vi "Constructor.vi"(8 "error in (no error)":errorcluster, 11 "Singleton.lvclass In":refnum<class "Singleton.lvclass">) -> (0 "error out":errorcluster, 3 "SingletonDVR Out":refnum<data-value>)   [LabVIEW 2013, in "Singleton.lvclass"]
uses:
  Singleton.lvclass
  Singleton.lvclass/Singleton.ctl
panel:
  # "SingletonConstructor"
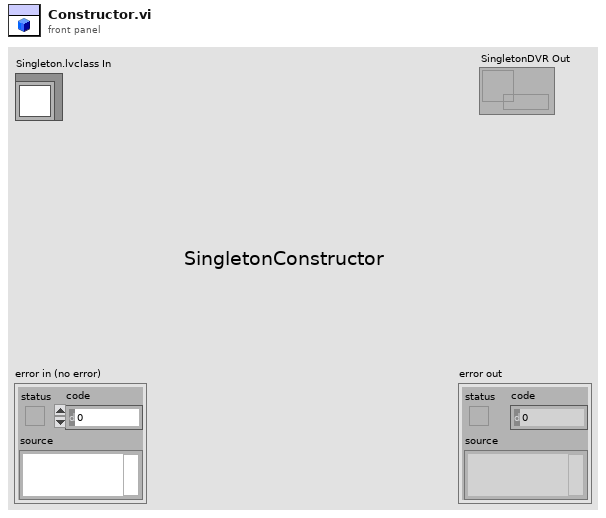
[diagram p1: front panel]
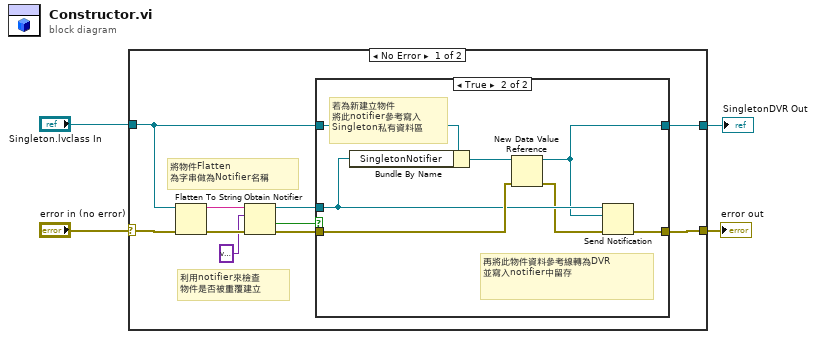
[diagram p0: block diagram]
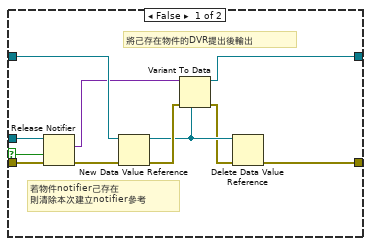
[diagram p2: hidden frame]
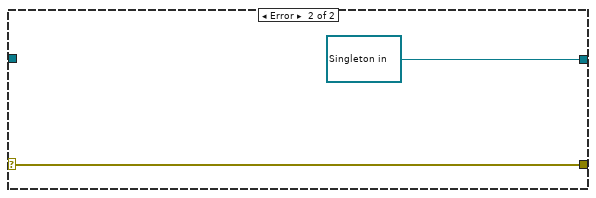
[diagram p3: hidden frame]
diagram:
  n1 = case shown="No Error" "error in (no error)" {
    selector: "error in (no error)" -> [w10 w34]
    tunnel: [w5 w34] -> w3
    tunnel: "Singleton.lvclass In" -> [w6 _]
    tunnel: [w8 refnum<data-value> refnum ("data value reference")] -> w1
    frame No Error {
      # "利用notifier來檢查\n物件是否被重覆建立"
      # "將物件Flatten\n為字串做為Notifier名稱"
      n2 = Flatten To String(anything=w6, error in (no error)=w10) -> (data string=w13:string, error out=w14:errorcluster)  [unwired: 2 in, 1 out]
      n3 = Obtain Notifier(name (unnamed)=w13, notification data type=variant ("DataVariant"), error in (no error)=w14) -> (notifier out=w11:refnum<notifier>, created new?=w12:bool, error out=w9:errorcluster)  [unwired: 1 in]
      n4 = case shown="True" w12 {
        selector: w12 -> [w25 _]
        tunnel: w11 -> [w23 w29]
        tunnel: w6 -> [w22 w32]
        tunnel: w9 -> [w24 w30]
        tunnel: [w15 w27] -> w8
        tunnel: [w16 w26] -> w5
        frame False {
          # "將己存在物件的DVR提出後輸出"
          # "若物件notifier己存在\n則清除本次建立notifier參考"
          n5 = Release Notifier(notifier=w23, force destroy? (F)=w25, error in (no error)=w24) -> (last notification=w18:variant, error out=w21:errorcluster)  [unwired: 1 out]
          n6 = New Data Value Reference(data value=w22, error in=w21) -> (data value reference=w19:refnum<data-value>, error out=w20:errorcluster)
          n7 = Variant To Data(error in=w20, type=w19, Variant=w18) -> (data=w15:refnum<data-value>, error out=w17:errorcluster)
          n8 = Delete Data Value Reference(data value reference=w19, error in=w17) -> (error out=w16:errorcluster)  [unwired: 1 out]
        }
        frame True {
          # "再將此物件資料參考線轉為DVR\n並寫入notifier中留存"
          # "若為新建立物件\n將此notifier參考寫入\nSingleton私有資料區"
          n9 = Bundle By Name(cluster=w32, "SingletonNotifier"=w29) -> (w31:refnum<class "Singleton.lvclass">)
          n10 = New Data Value Reference(data value=w31, error in=w30) -> (data value reference=w27:refnum<data-value>, error out=w28:errorcluster)
          n11 = Send Notification(notification=w27, notifier=w29, error in (no error)=w28) -> (error out=w26:errorcluster)  [unwired: 1 out]
        }
      }
    }
    frame Error {
    }
  }
  "error out" <- w3
  "SingletonDVR Out" <- w1
